vi "Get Remote Connection Options.vi"(8 "error in":errorcluster, 10 "session name":string="test_sess", 11 "provided interface":string) -> (0 "error out":errorcluster, 3 "remote connection options":T1)   [LabVIEW 2020, in "MeasurementServerTests.lvlib"]
uses:
  MeasurementServerTests.lvlib
  Runtime/MeasurementLink Instrument/IInstrument/Remote Connection Options.ctl
  Runtime/MeasurementLink gRPC Utilities/TypeDefs/Service Location FGV Action.ctl
  Runtime/MeasurementLink Discovery Client/RPC Messages/ni_measurementlink_discovery_v1_ResolveServiceRequest.ctl
  Runtime/MeasurementLink Discovery Client/MeasurementLink Discovery Client.lvlib
  Runtime/MeasurementLink Instrument/IInstrument/IInstrument.lvclass
  Runtime/MeasurementLink gRPC Utilities/MeasurementLink gRPC Utilities.lvlib
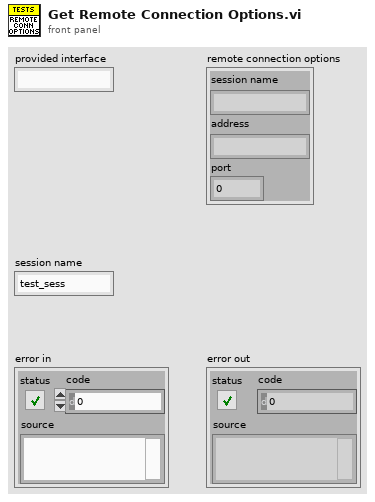
[diagram p1: front panel]
types:
  T1 = typedef "MeasurementLink Instrument.lvlib/IInstrument.lvclass/Remote Connection Options.ctl" = cluster{"session name":string, "address":string, "port":u32}
  T2 = typedef "MeasurementLink Discovery Client.lvlib/ni_measurementlink_discovery_v1_ResolveServiceRequest.ctl" = cluster{"provided_interface":string, "service_class":string}
  T3 = typedef "MeasurementLink gRPC Utilities.lvlib/Service Location FGV Action.ctl" = enum16{"Get Service Location", "Clear Cache"}
  T4 = typedef "MeasurementLink Discovery Client.lvlib/ni_measurementlink_discovery_v1_ServiceLocation.ctl" = cluster{"location":string, "insecure_port":string, "ssl_authenticated_port":string}
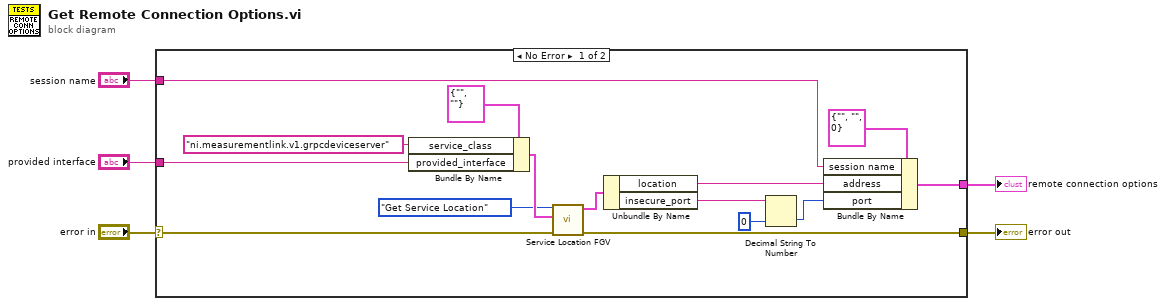
[diagram p0: block diagram]
diagram:
  n1 = case shown="No Error" "error in" {
    selector: "error in" -> [w11 w21]
    tunnel: [w20 _] -> w5
    tunnel: [w12 w21] -> w4
    tunnel: "provided interface" -> [w10 _]
    tunnel: "session name" -> [w6 _]
    frame No Error {
      n2 = Bundle By Name(cluster=T2 {"provided_interface"="", "service_class"=""} ("Resolve Service Request"), "service_class"="ni.measurementlink.v1.grpcdeviceserver", "provided_interface"=w10) -> (w13:T2)
      n3 = call "Service Location FGV.vi"("error in"=w11, "Resolve Service Request"=w13, "Action"=Service_Location_FGV_Action."Get Service Location") -> ("error out"=w12:errorcluster, "Service Location"=w14:T4)  [unwired: 7 in]
      n4 = Unbundle By Name(w14) -> ("location"=w16:string, "insecure_port"=w17:string)
      n5 = Decimal String To Number(string=w17, default (0L)=u32 0 ("default (0 I32)")) -> (number=w18:u32)  [unwired: 1 in, 1 out]
      n6 = Bundle By Name(cluster=T1 {"session name"="", "address"="", "port"=0} ("remote connection options"), "session name"=w6, "address"=w16, "port"=w18) -> (w20:T1)
    }
    frame Error {
    }
  }
  "remote connection options" <- w5
  "error out" <- w4
